vi "HW1 Calculator.vi"() -> ()   [LabVIEW 2023]
uses:
  <vilib>/gmath/NI_Gmath.lvlib
panel:
  in  "1/x":bool
  out "Save 2":ext
  out "Save1":ext
  in  "Save 2":bool
  in  "Save 1":bool
  out "Answer":ext
  out "運行時間":string
  in  "stop":bool
  out "Display":string
  in  ")":bool
  in  "(":bool
  in  "=":bool
  in  "+":bool
  in  ".":bool
  in  "+/-":bool
  in  "0":bool
  in  "Backspace":bool
  in  "CE":bool
  in  "C":bool
  in  "SQRT":bool
  in  "-":bool
  in  "*":bool
  in  "/":bool
  in  "9":bool
  in  "8":bool
  in  "7":bool
  in  "6":bool
  in  "5":bool
  in  "4":bool
  in  "3":bool
  in  "2":bool
  in  "1":bool
  out "current time":timestamp format="%<%I:%M:%S %p\n%x>T"
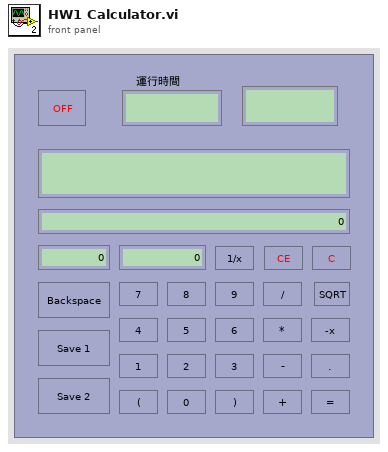
[diagram p1: front panel]
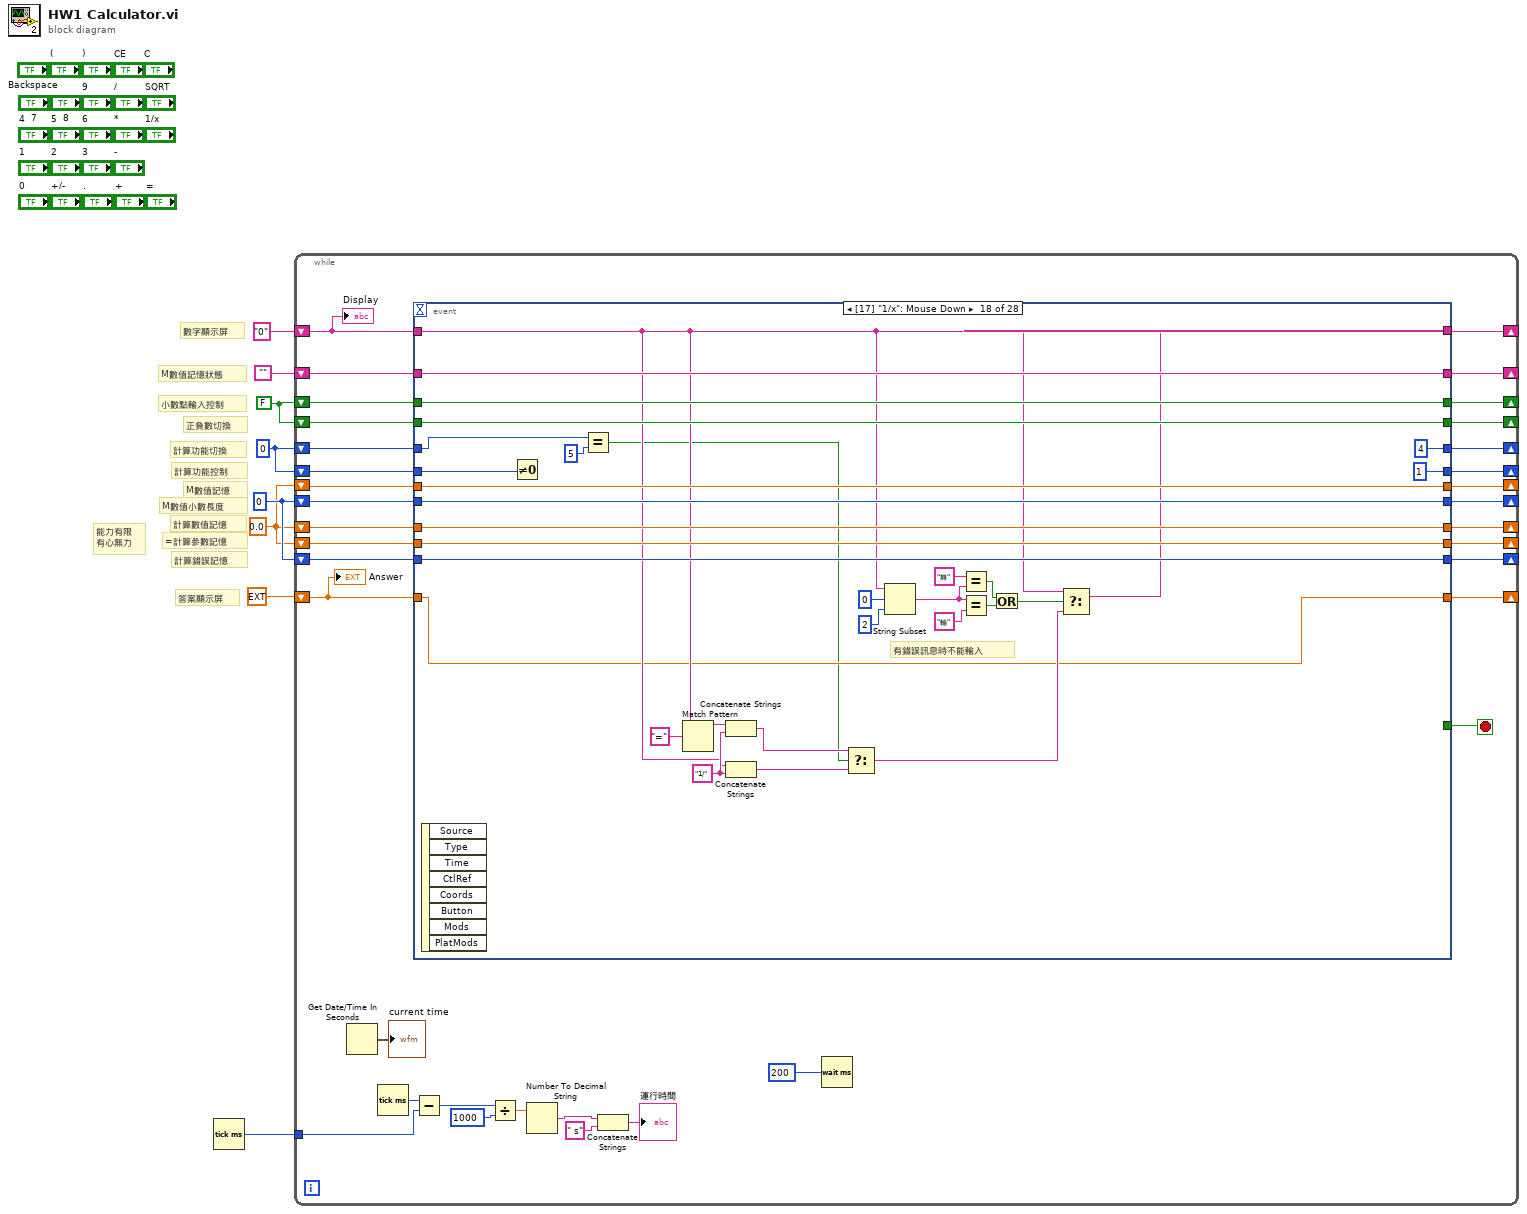
[diagram p0: block diagram]
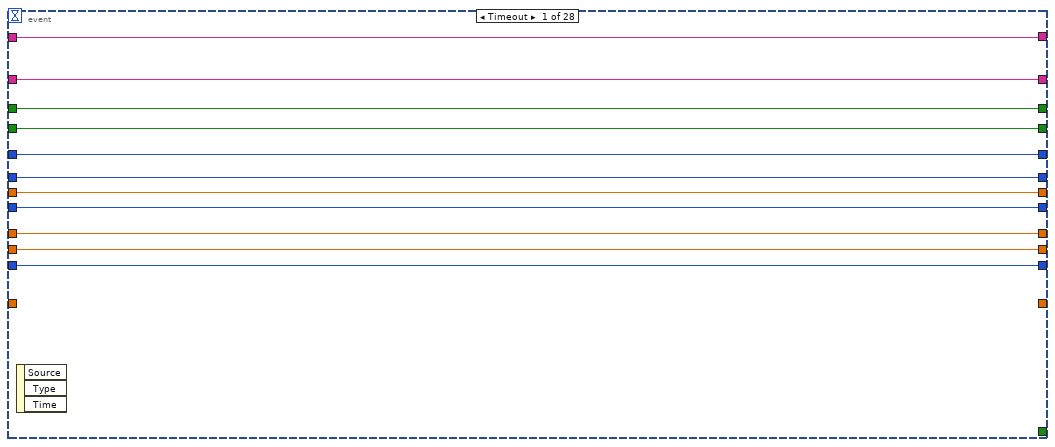
[diagram p2: hidden frame]
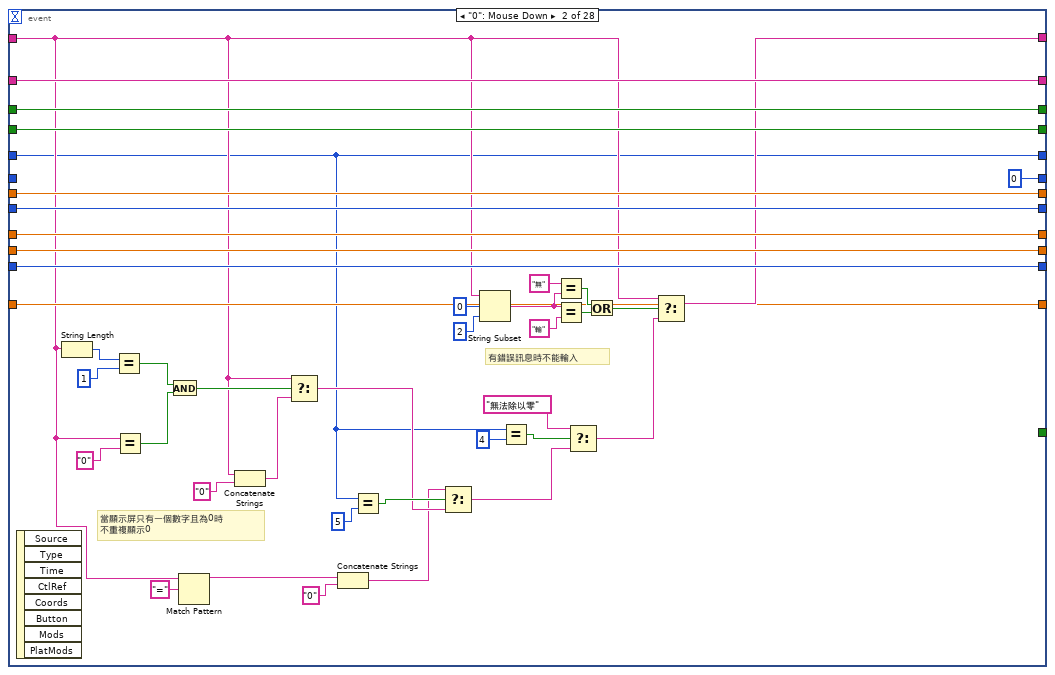
[diagram p3: hidden frame]
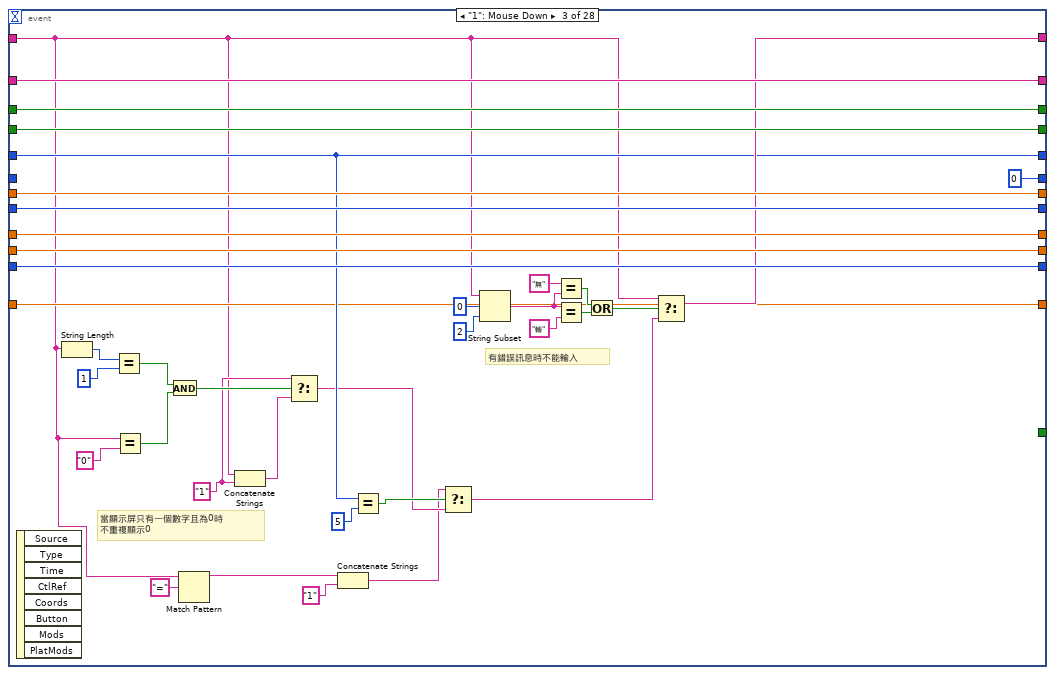
[diagram p4: hidden frame]
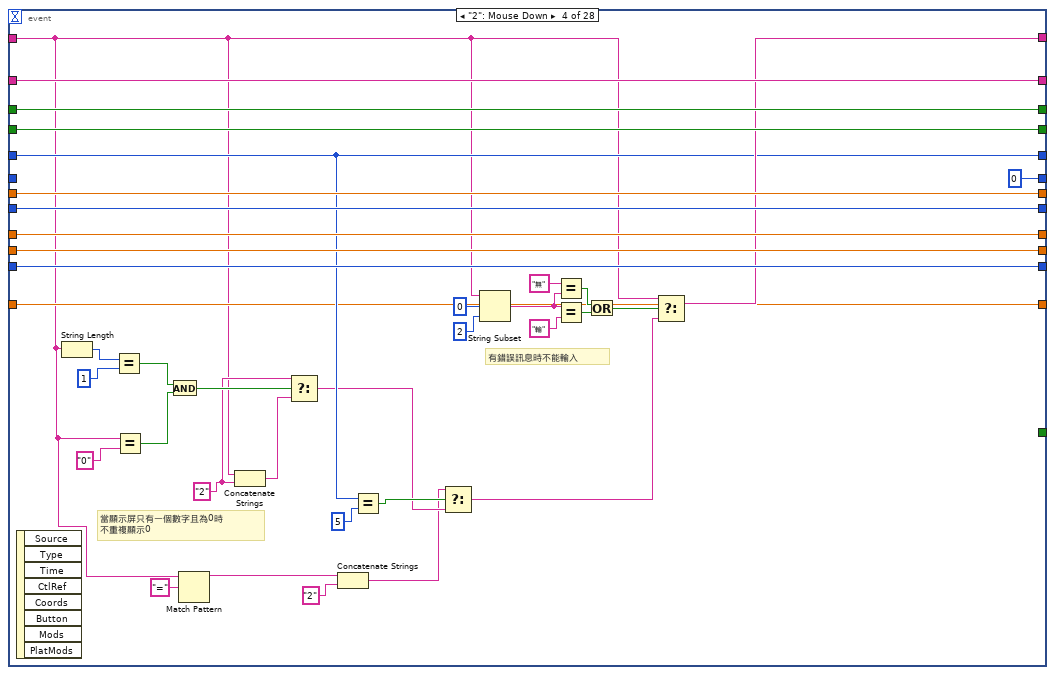
[diagram p5: hidden frame]
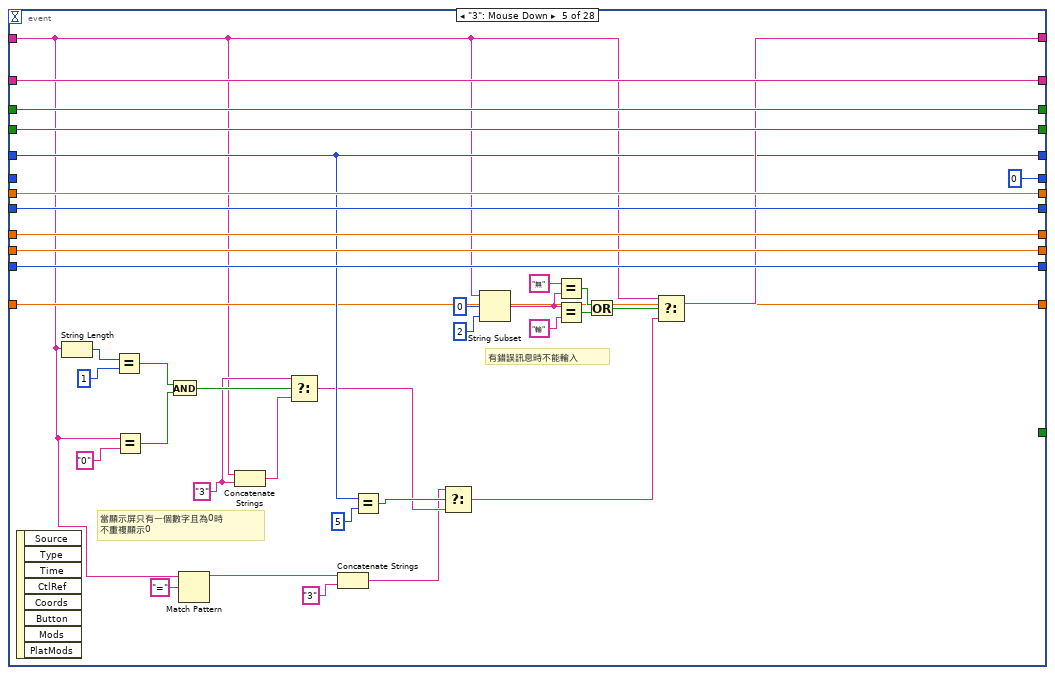
[diagram p6: hidden frame]
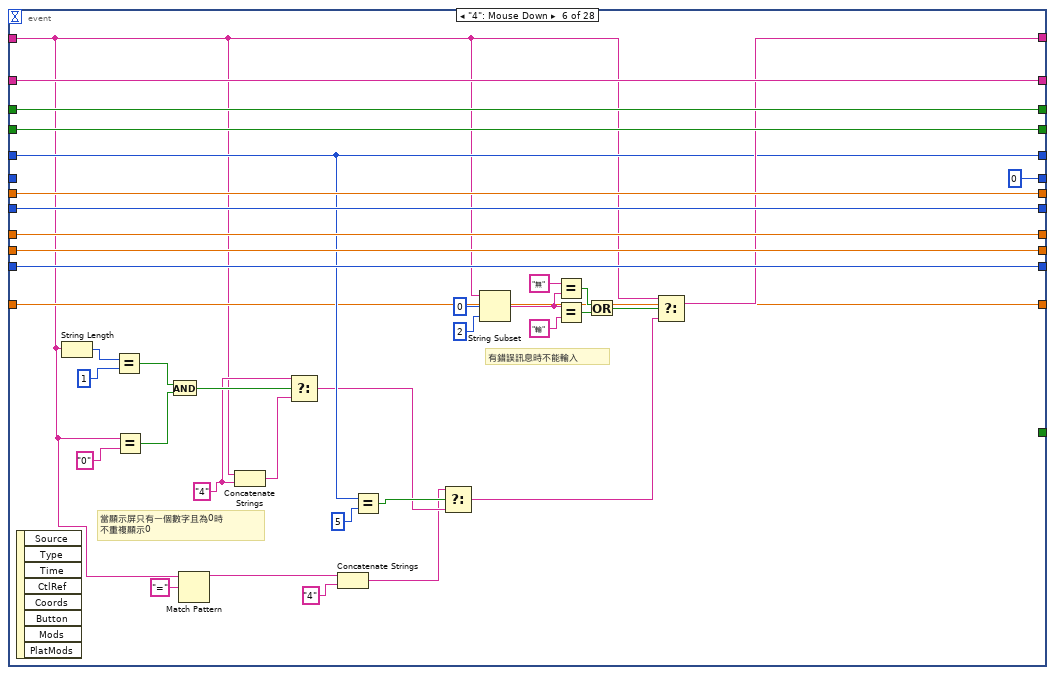
[diagram p7: hidden frame]
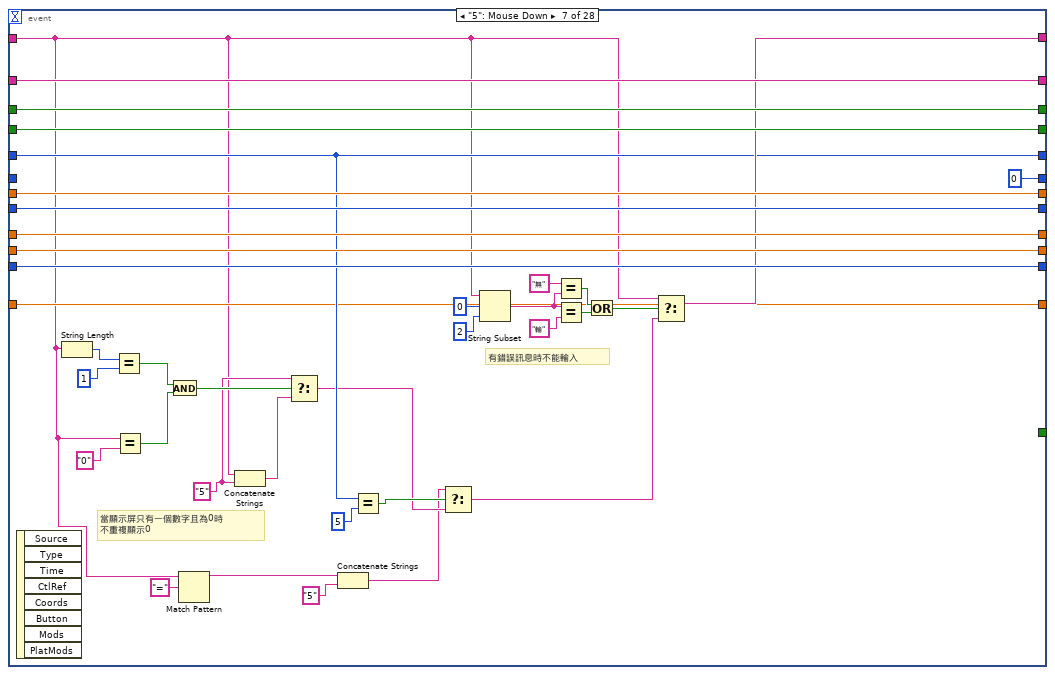
[diagram p8: hidden frame]
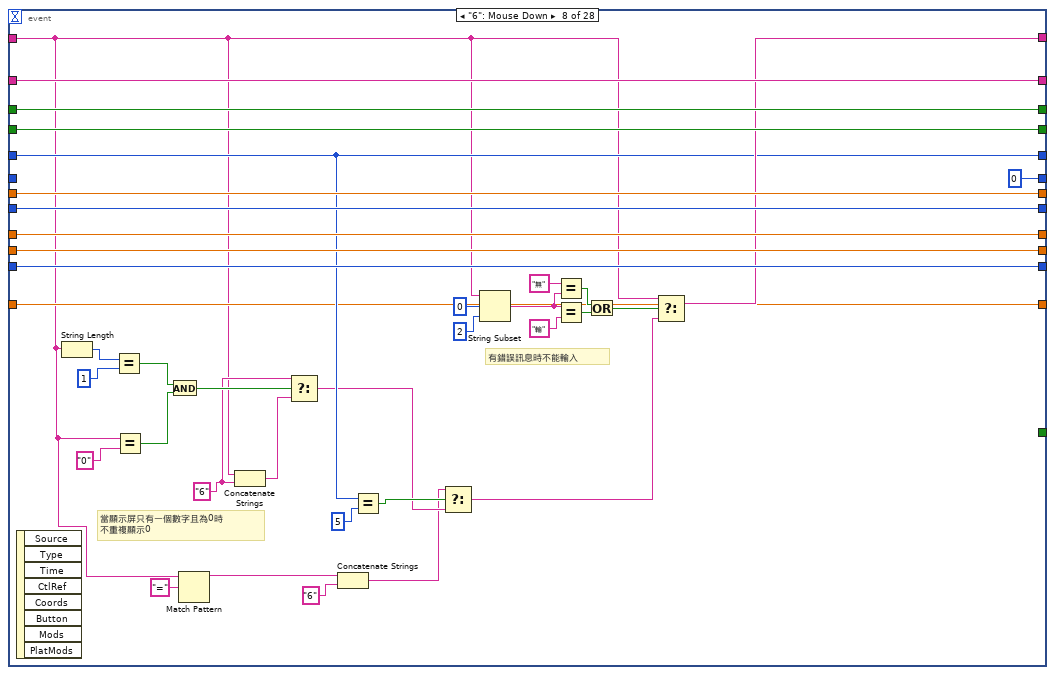
[diagram p9: hidden frame]
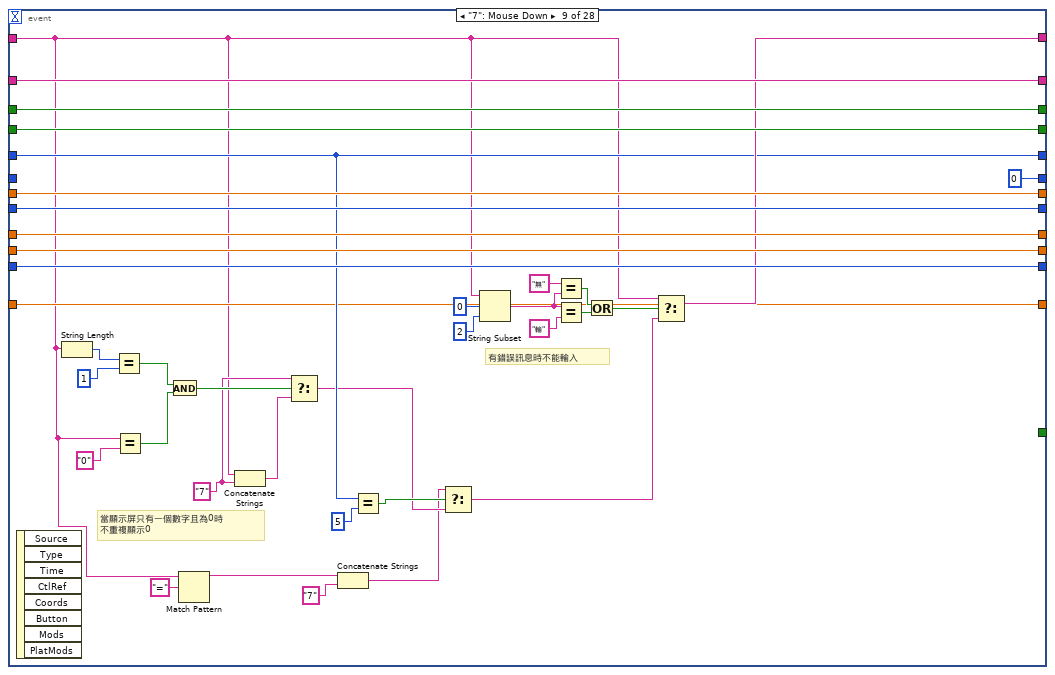
[diagram p10: hidden frame]
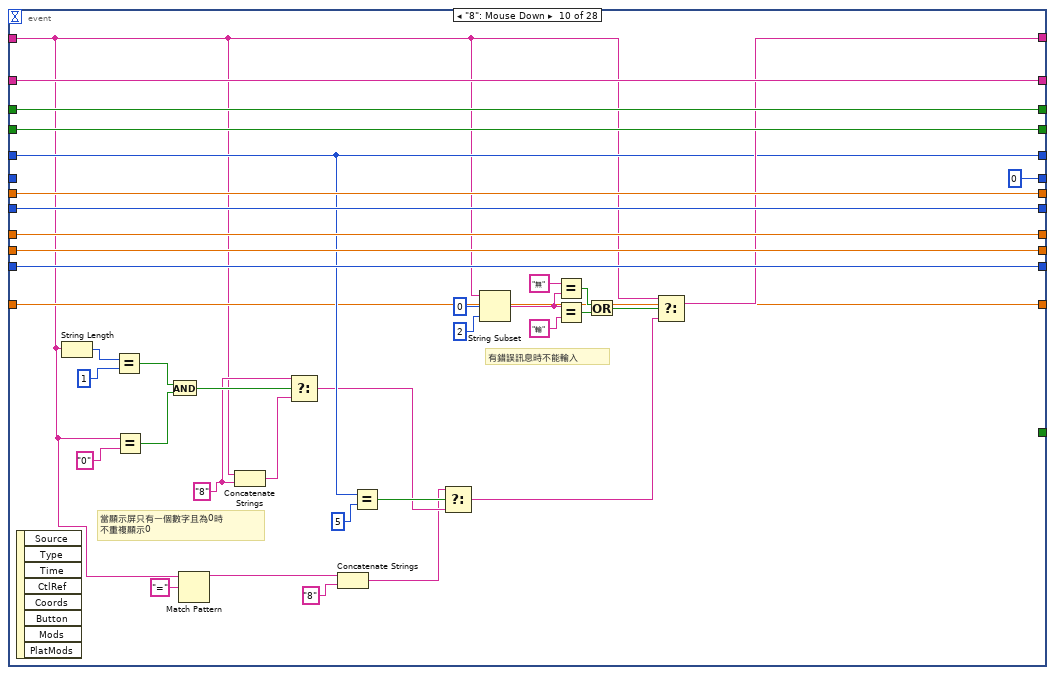
[diagram p11: hidden frame]
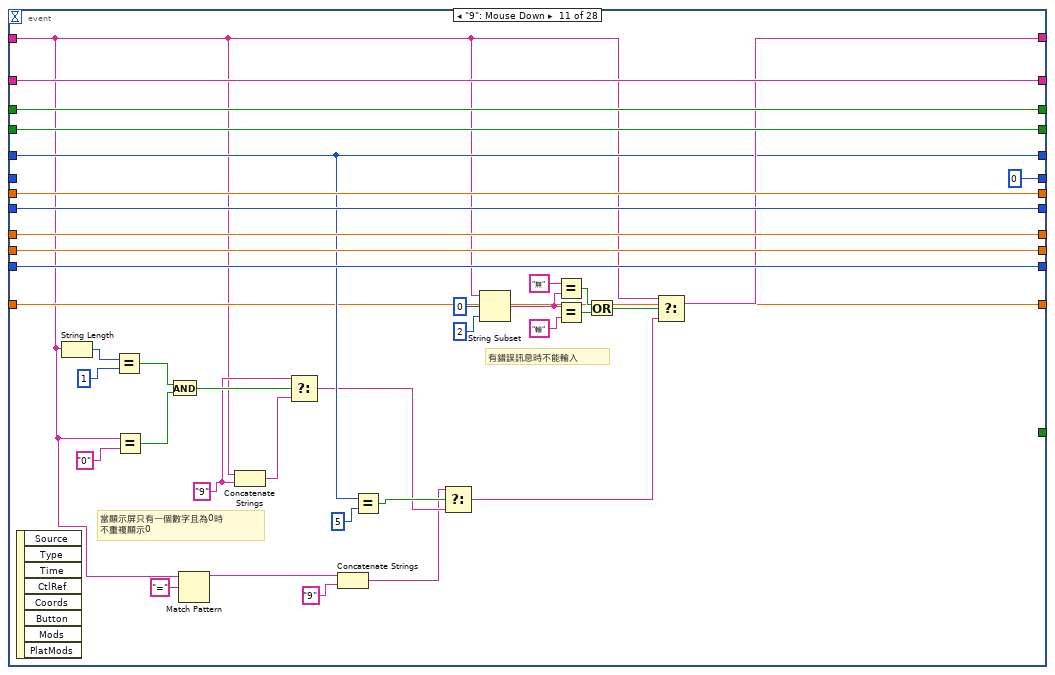
[diagram p12: hidden frame]
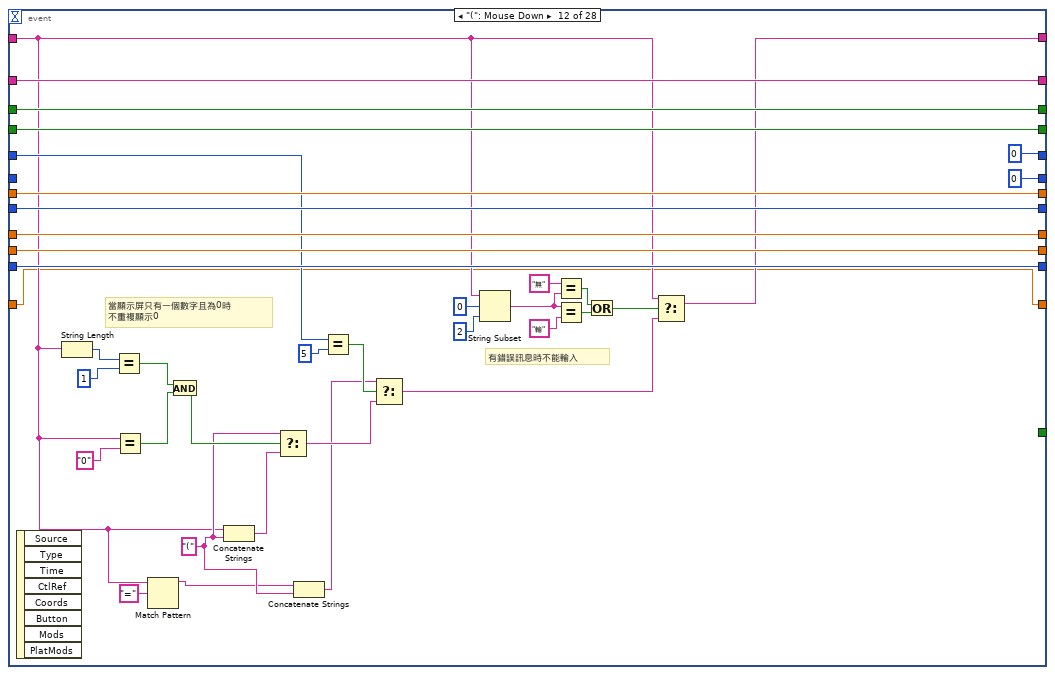
[diagram p13: hidden frame]
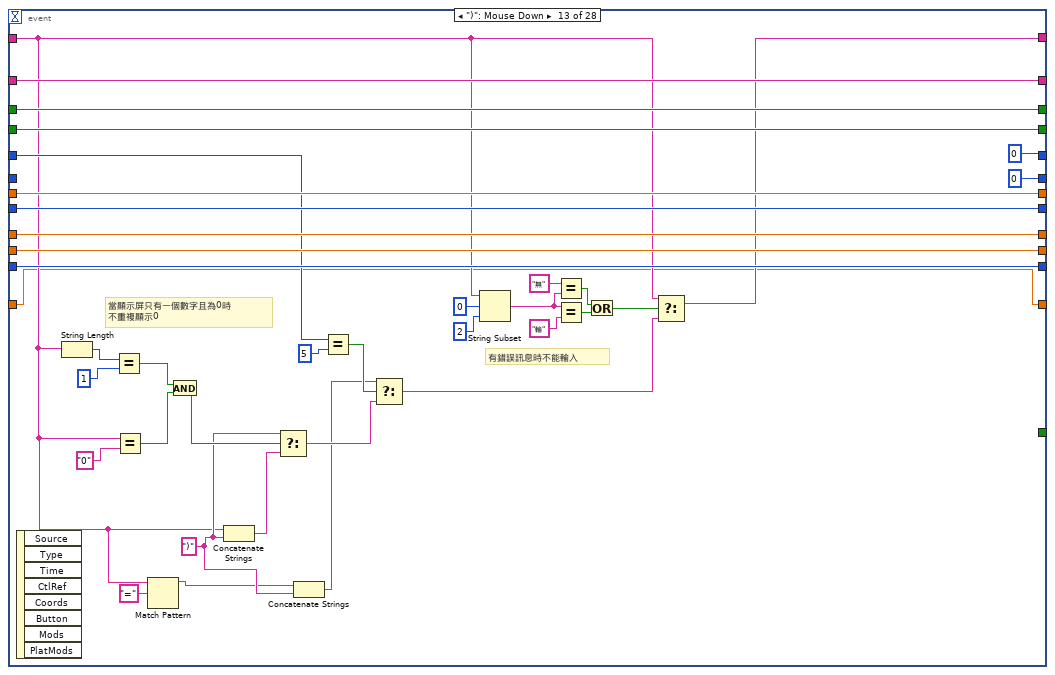
[diagram p14: hidden frame]
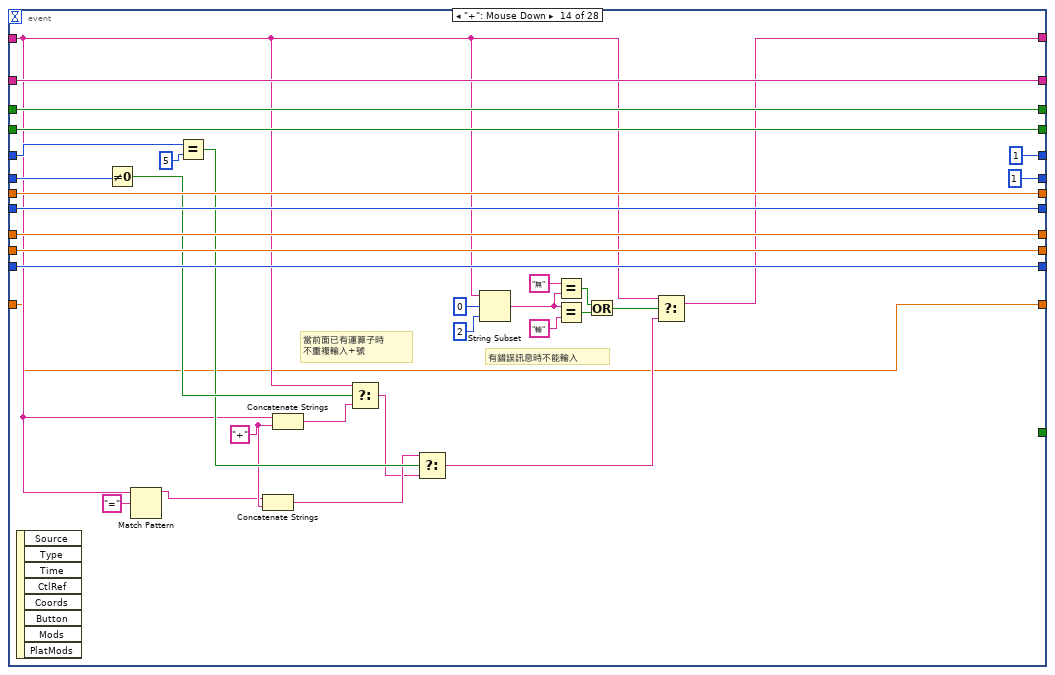
[diagram p15: hidden frame]
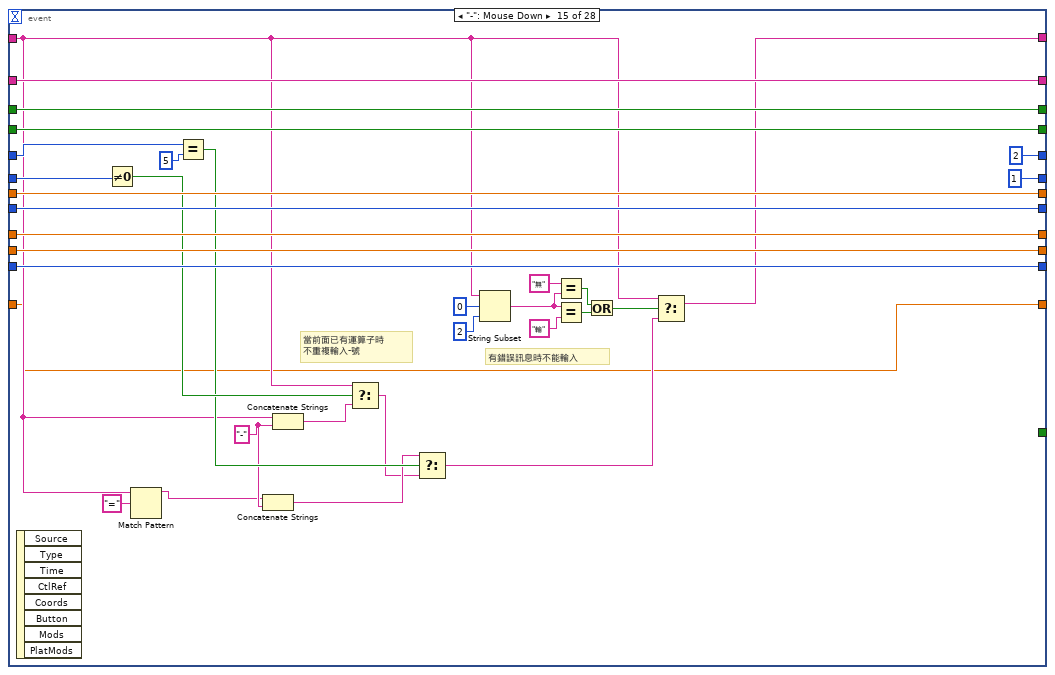
[diagram p16: hidden frame]
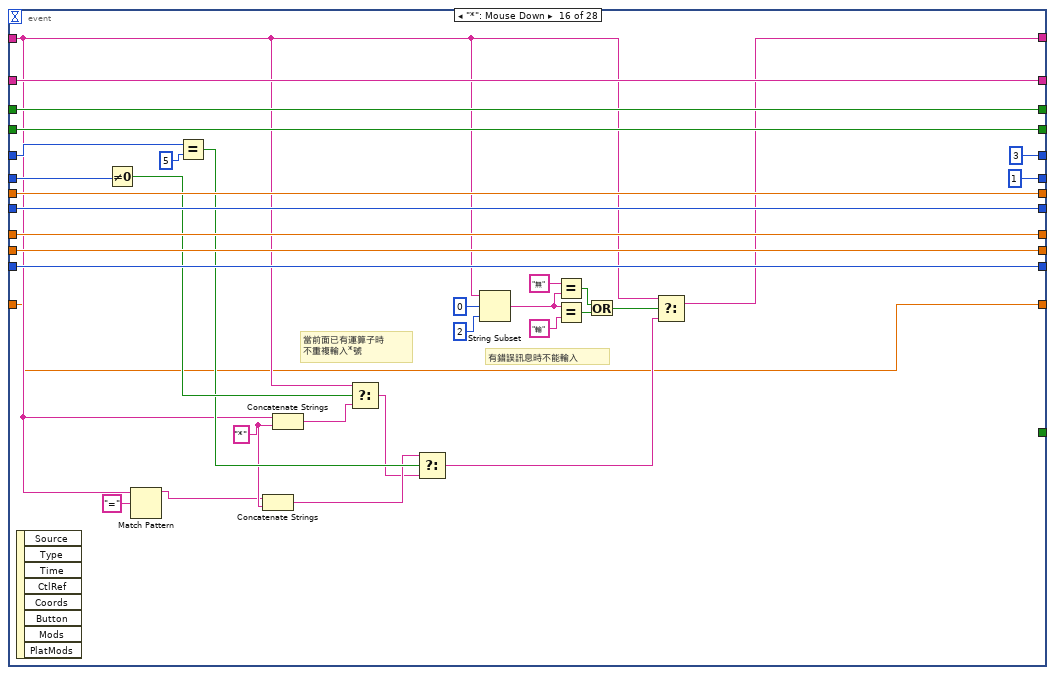
[diagram p17: hidden frame]
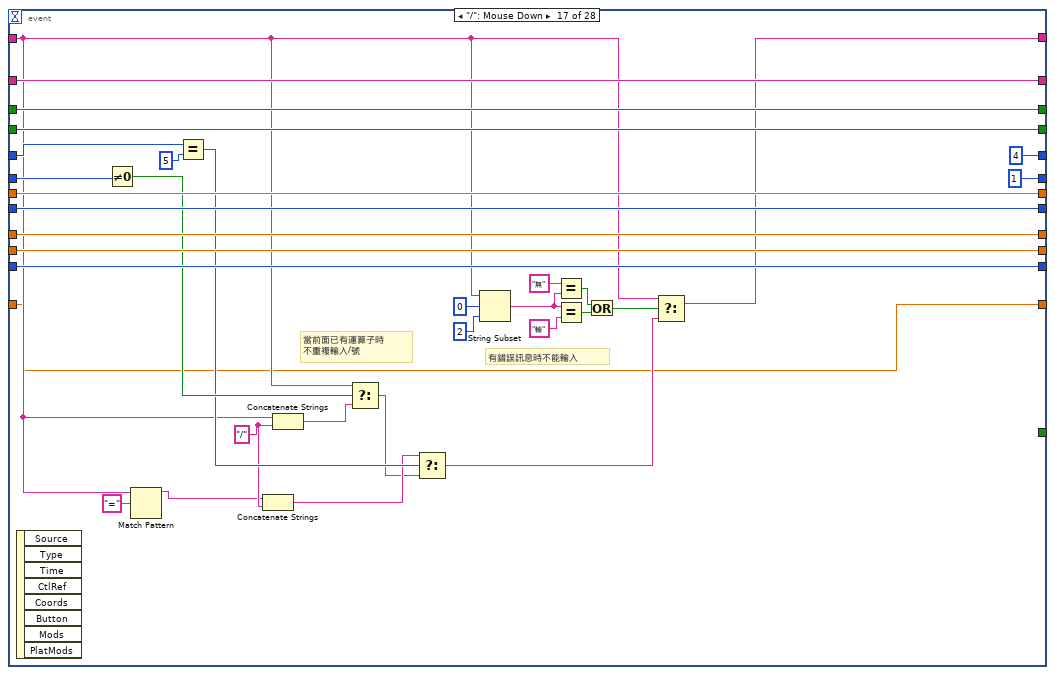
[diagram p18: hidden frame]
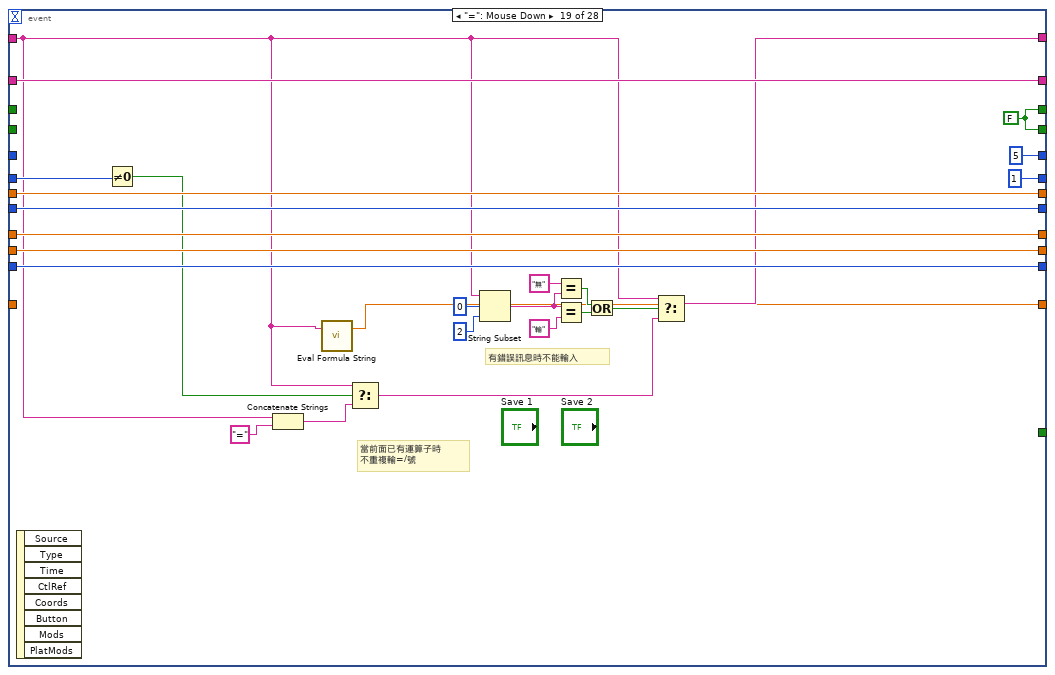
[diagram p19: hidden frame]
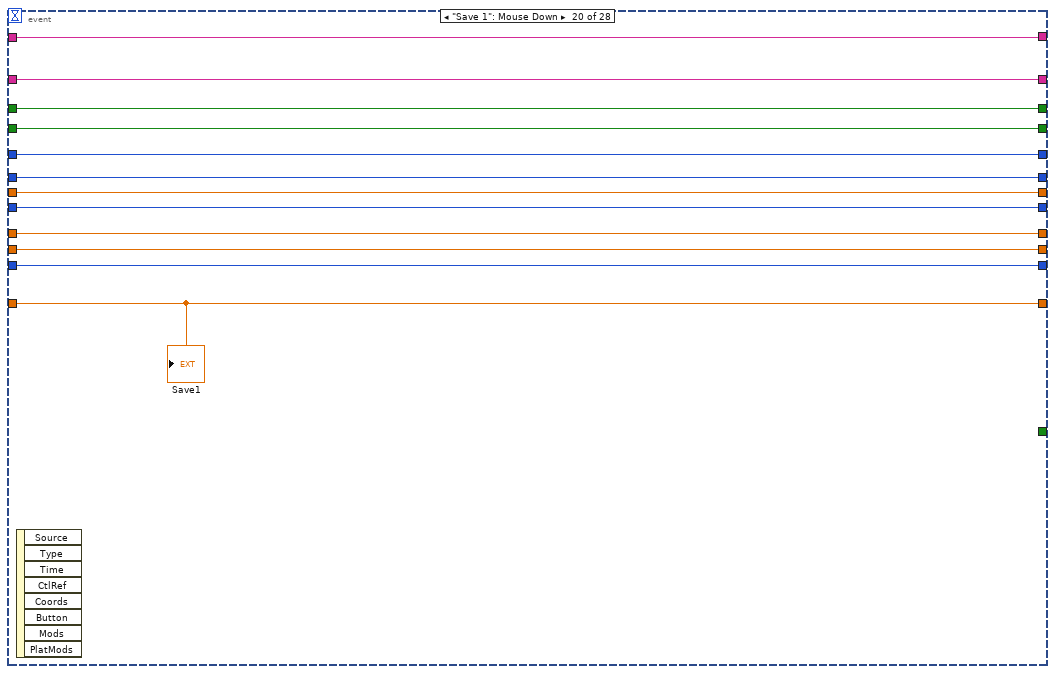
[diagram p20: hidden frame]
diagram:
  w3 = 0.0
  w4 = 0
  w5 = 0
  w6 = FALSE
  # "能力有限\n有心無力"
  # "答案顯示屏"
  # "M數值小數長度"
  # "計算錯誤記憶"
  # "=計算參數記憶"
  # "計算數值記憶"
  # "M數值記憶"
  # "計算功能控制"
  # "計算功能切換"
  # "正負數切換"
  # "小數點輸入控制"
  # "M數值記憶狀態"
  # "數字顯示屏"
  n1 = Tick Count (ms)() -> (millisecond timer value=w2:u32)
  n2 = while {
    shift-right: [w43] -> _
    shift-left: "0" -> [w24]
    shift-right: [w42] -> _
    shift-left: "" -> [w23]
    shift-right: [w40] -> _
    shift-left: w6 -> [w41]
    shift-right: [w38] -> _
    shift-left: w6 -> [w39]
    shift-right: [w37] -> _
    shift-left: w5 -> [w22]
    shift-right: [w35] -> _
    shift-left: w5 -> [w36]
    shift-right: [w27] -> _
    shift-left: w3 -> [w28]
    shift-right: [w33] -> _
    shift-left: w4 -> [w34]
    shift-right: [w29] -> _
    shift-left: w3 -> [w30]
    shift-right: [w25] -> _
    shift-left: w3 -> [w26]
    shift-right: [w31] -> _
    shift-left: w4 -> [w32]
    tunnel: w2 -> [w20]
    shift-right: [w12] -> _
    shift-left: ext 0.0 -> [w11]
    stop <- w21 stop-if-true
    n3 = Get Date/Time In Seconds() -> (seconds since 1Jan1904=→"current time":timestamp)
    n4 = Tick Count (ms)() -> (millisecond timer value=w19:u32)
    n5 = event shown="[17] \"1/x\": Mouse Down" {
      selector: _ -> [_ _ _ _ _ _ _ _ _ _ _ _ _ _ _ _ _ _ _ _ _ _ _ _ _ _ _ _]
      dyn-events: _ -> [_ _ _ _ _ _ _ _ _ _ _ _ _ _ _ _ _ _ _ _ _ _ _ _ _ _ _ _]
      timeout: _ -> [_ _ _ _ _ _ _ _ _ _ _ _ _ _ _ _ _ _ _ _ _ _ _ _ _ _ _ _]
      tunnel: w24 -> [w54 w64 w98 w135 w172 w209 w246 w283 w320 w357 w394 w432 w469 w506 w539 w572 w605 w640 w669 w702 w714 w724 w765 w802 _ w869 w881 _]
      tunnel: [w54 w70 w108 w145 w182 w219 w256 w293 w330 w367 w404 w441 w478 w518 w551 w584 w617 w648 w675 w702 w714 w740 w785 w824 "0" w868 w893 _] -> w43
      tunnel: w23 -> [w53 w95 w132 w169 w206 w243 w280 w317 w354 w391 w428 w465 w502 w535 w568 w601 w634 w665 w690 w701 w713 w760 w800 w839 w847 w874 w894 _]
      tunnel: [w53 w95 w132 w169 w206 w243 w280 w317 w354 w391 w428 w465 w502 w535 w568 w601 w634 w665 w690 w701 w713 w760 w800 w839 w847 w874 w894 _] -> w42
      tunnel: w41 -> [w52 w94 w131 w168 w205 w242 w279 w316 w353 w390 w427 w464 w501 w534 w567 w600 w633 w664 _ w700 w712 w759 w770 w810 _ w867 w896 _]
      tunnel: [w52 w94 w131 w168 w205 w242 w279 w316 w353 w390 w427 w464 w501 w534 w567 w600 w633 w664 w666 w700 w712 w759 w769 w820 w848 w866 w896 _] -> w40
      tunnel: w39 -> [w51 w93 w130 w167 w204 w241 w278 w315 w352 w389 w426 w463 w500 w533 w566 w599 w632 w663 _ w699 w711 w736 w774 w838 _ w864 w895 _]
      tunnel: [w51 w93 w130 w167 w204 w241 w278 w315 w352 w389 w426 w463 w500 w533 w566 w599 w632 w663 w666 w699 w711 w729 w768 w838 w848 w863 w895 _] -> w38
      tunnel: w22 -> [w50 w59 w106 w143 w180 w217 w254 w291 w328 w365 w402 w440 w477 w512 w545 w578 w611 w644 _ w698 w710 w721 _ w815 _ w861 w883 _]
      tunnel: [w50 w59 w106 w143 w180 w217 w254 w291 w328 w365 w402 0 0 1 2 3 4 4 5 w698 w710 0 0 0 w840 w859 w885 _] -> w37
      tunnel: w36 -> [w49 _ _ _ _ _ _ _ _ _ _ _ _ w517 w550 w583 w616 w647 w673 w697 w709 w734 w779 w819 _ w860 _ _]
      tunnel: [w49 0 0 0 0 0 0 0 0 0 0 0 0 1 1 1 1 1 1 w697 w709 0 w779 0 w840 w858 w885 _] -> w35
      tunnel: w34 -> [w48 w91 w128 w165 w202 w239 w276 w313 w350 w387 w424 w461 w498 w531 w564 w597 w630 w661 w688 w695 w707 w757 w798 w836 w845 w872 w911 _]
      tunnel: [w48 w91 w128 w165 w202 w239 w276 w313 w350 w387 w424 w461 w498 w531 w564 w597 w630 w661 w688 w695 w707 w757 w798 w836 w845 w872 w911 _] -> w33
      tunnel: w32 -> [w47 w88 w125 w162 w199 w236 w273 w310 w347 w384 w421 w458 w495 w528 w561 w594 w627 w658 w685 w692 w704 w754 w795 w833 w842 w853 w908 _]
      tunnel: [w47 w88 w125 w162 w199 w236 w273 w310 w347 w384 w421 w458 w495 w528 w561 w594 w627 w658 w685 w692 w704 w754 w795 w833 w842 w852 w908 _] -> w31
      tunnel: w30 -> [w46 w90 w127 w164 w201 w238 w275 w312 w349 w386 w423 w460 w497 w530 w563 w596 w629 w660 w687 w694 w706 w756 w797 w835 w844 w856 w910 _]
      tunnel: [w46 w90 w127 w164 w201 w238 w275 w312 w349 w386 w423 w460 w497 w530 w563 w596 w629 w660 w687 w694 w706 w756 w797 w835 w844 w854 w910 _] -> w29
      tunnel: w28 -> [w45 w92 w129 w166 w203 w240 w277 w314 w351 w388 w425 w462 w499 w532 w565 w598 w631 w662 w689 w696 w708 w758 w799 w837 w846 w873 w912 _]
      tunnel: [w45 w92 w129 w166 w203 w240 w277 w314 w351 w388 w425 w462 w499 w532 w565 w598 w631 w662 w689 w696 w708 w758 w799 w837 w846 w873 w912 _] -> w27
      tunnel: w26 -> [w44 w89 w126 w163 w200 w237 w274 w311 w348 w385 w422 w459 w496 w529 w562 w595 w628 w659 w686 w693 w705 w755 w796 w834 w843 w855 w909 _]
      tunnel: [w44 w89 w126 w163 w200 w237 w274 w311 w348 w385 w422 w459 w496 w529 w562 w595 w628 w659 w686 w693 w705 w755 w796 w834 w843 w850 w909 _] -> w25
      tunnel: [_ _ _ _ _ _ _ _ _ _ _ _ _ _ _ _ _ _ _ _ _ _ _ _ _ _ _ w913] -> w21
      tunnel: [_ w65 w100 w137 w174 w211 w248 w285 w322 w359 w396 w429 w466 w503 w536 w569 w602 w637 w667 w691 w703 _ w761 _ w841 w850 w876 _] -> w12
      tunnel: w11 -> [_ w65 w100 w137 w174 w211 w248 w285 w322 w359 w396 w429 w466 w503 w536 w569 w602 w637 _ w691 w703 w719 w761 _ w841 _ w876 _]
      event Timeout {
        n6 = event-data() -> ()  [unwired: 1 in, 3 out]
      }
      event "0": Mouse Down {
        # "有錯誤訊息時不能輸入"
        # "當顯示屏只有一個數字且為0時\n不重複顯示0"
        n7 = event-data() -> ()  [unwired: 1 in, 8 out]
        n8 = String Length(string=w64) -> (length=w85:i32)
        n9 = Equal?(x=w85, y=1) -> (x = y?=w83:bool)
        n10 = Equal?(x=w64, y="0") -> (x = y?=w82:bool)
        n11 = And(x=w83, y=w82) -> (x .and. y?=w80:bool)
        n12 = Match Pattern(string=w64, regular expression="=") -> (before substring=w62:string)  [unwired: 1 in, 3 out]
        n13 = Concatenate Strings(w64, "0") -> (w79:string)
        n14 = Select(t=w64, s=w80, f=w79) -> (s? t:f=w67:string)
        n15 = Concatenate Strings(w62, "0") -> (w61:string)
        n16 = Equal?(x=w59, y=5) -> (x = y?=w68:bool)
        n17 = Select(t=w61, s=w68, f=w67) -> (s? t:f=w58:string)
        n18 = String Subset(string=w64, offset (0)=0, length (rest)=2) -> (substring=w74:string)
        n19 = Equal?(x=w59, y=4) -> (x = y?=w57:bool)
        n20 = Equal?(x="無", y=w74) -> (x = y?=w73:bool)
        n21 = Equal?(x=w74, y="輸") -> (x = y?=w72:bool)
        n22 = Select(t="無法除以零", s=w57, f=w58) -> (s? t:f=w55:string)
        n23 = Or(x=w73, y=w72) -> (x .or. y?=w71:bool)
        n24 = Select(t=w64, s=w71, f=w55) -> (s? t:f=w70:string)
      }
      event "1": Mouse Down {
        w99 = "1"
        # "有錯誤訊息時不能輸入"
        # "當顯示屏只有一個數字且為0時\n不重複顯示0"
        n25 = event-data() -> ()  [unwired: 1 in, 8 out]
        n26 = String Length(string=w98) -> (length=w122:i32)
        n27 = Equal?(x=w122, y=1) -> (x = y?=w120:bool)
        n28 = Equal?(x=w98, y="0") -> (x = y?=w119:bool)
        n29 = And(x=w120, y=w119) -> (x .and. y?=w118:bool)
        n30 = Match Pattern(string=w98, regular expression="=") -> (before substring=w96:string)  [unwired: 1 in, 3 out]
        n31 = Concatenate Strings(w98, w99) -> (w117:string)
        n32 = Select(t=w99, s=w118, f=w117) -> (s? t:f=w104:string)
        n33 = Concatenate Strings(w96, "1") -> (w102:string)
        n34 = Equal?(x=w106, y=5) -> (x = y?=w105:bool)
        n35 = Select(t=w102, s=w105, f=w104) -> (s? t:f=w101:string)
        n36 = String Subset(string=w98, offset (0)=0, length (rest)=2) -> (substring=w112:string)
        n37 = Equal?(x="無", y=w112) -> (x = y?=w111:bool)
        n38 = Equal?(x=w112, y="輸") -> (x = y?=w110:bool)
        n39 = Or(x=w111, y=w110) -> (x .or. y?=w109:bool)
        n40 = Select(t=w98, s=w109, f=w101) -> (s? t:f=w108:string)
      }
      event "2": Mouse Down {
        w136 = "2"
        # "有錯誤訊息時不能輸入"
        # "當顯示屏只有一個數字且為0時\n不重複顯示0"
        n41 = event-data() -> ()  [unwired: 1 in, 8 out]
        n42 = String Length(string=w135) -> (length=w159:i32)
        n43 = Equal?(x=w159, y=1) -> (x = y?=w157:bool)
        n44 = Equal?(x=w135, y="0") -> (x = y?=w156:bool)
        n45 = And(x=w157, y=w156) -> (x .and. y?=w155:bool)
        n46 = Match Pattern(string=w135, regular expression="=") -> (before substring=w133:string)  [unwired: 1 in, 3 out]
        n47 = Concatenate Strings(w135, w136) -> (w154:string)
        n48 = Select(t=w136, s=w155, f=w154) -> (s? t:f=w141:string)
        n49 = Concatenate Strings(w133, "2") -> (w139:string)
        n50 = Equal?(x=w143, y=5) -> (x = y?=w142:bool)
        n51 = Select(t=w139, s=w142, f=w141) -> (s? t:f=w138:string)
        n52 = String Subset(string=w135, offset (0)=0, length (rest)=2) -> (substring=w149:string)
        n53 = Equal?(x="無", y=w149) -> (x = y?=w148:bool)
        n54 = Equal?(x=w149, y="輸") -> (x = y?=w147:bool)
        n55 = Or(x=w148, y=w147) -> (x .or. y?=w146:bool)
        n56 = Select(t=w135, s=w146, f=w138) -> (s? t:f=w145:string)
      }
      event "3": Mouse Down {
        w173 = "3"
        # "有錯誤訊息時不能輸入"
        # "當顯示屏只有一個數字且為0時\n不重複顯示0"
        n57 = event-data() -> ()  [unwired: 1 in, 8 out]
        n58 = String Length(string=w172) -> (length=w196:i32)
        n59 = Equal?(x=w196, y=1) -> (x = y?=w194:bool)
        n60 = Equal?(x=w172, y="0") -> (x = y?=w193:bool)
        n61 = And(x=w194, y=w193) -> (x .and. y?=w192:bool)
        n62 = Match Pattern(string=w172, regular expression="=") -> (before substring=w170:string)  [unwired: 1 in, 3 out]
        n63 = Concatenate Strings(w172, w173) -> (w191:string)
        n64 = Select(t=w173, s=w192, f=w191) -> (s? t:f=w178:string)
        n65 = Concatenate Strings(w170, "3") -> (w176:string)
        n66 = Equal?(x=w180, y=5) -> (x = y?=w179:bool)
        n67 = Select(t=w176, s=w179, f=w178) -> (s? t:f=w175:string)
        n68 = String Subset(string=w172, offset (0)=0, length (rest)=2) -> (substring=w186:string)
        n69 = Equal?(x="無", y=w186) -> (x = y?=w185:bool)
        n70 = Equal?(x=w186, y="輸") -> (x = y?=w184:bool)
        n71 = Or(x=w185, y=w184) -> (x .or. y?=w183:bool)
        n72 = Select(t=w172, s=w183, f=w175) -> (s? t:f=w182:string)
      }
      event "4": Mouse Down {
        w210 = "4"
        # "有錯誤訊息時不能輸入"
        # "當顯示屏只有一個數字且為0時\n不重複顯示0"
        n73 = event-data() -> ()  [unwired: 1 in, 8 out]
        n74 = String Length(string=w209) -> (length=w233:i32)
        n75 = Equal?(x=w233, y=1) -> (x = y?=w231:bool)
        n76 = Equal?(x=w209, y="0") -> (x = y?=w230:bool)
        n77 = And(x=w231, y=w230) -> (x .and. y?=w229:bool)
        n78 = Match Pattern(string=w209, regular expression="=") -> (before substring=w207:string)  [unwired: 1 in, 3 out]
        n79 = Concatenate Strings(w209, w210) -> (w228:string)
        n80 = Select(t=w210, s=w229, f=w228) -> (s? t:f=w215:string)
        n81 = Concatenate Strings(w207, "4") -> (w213:string)
        n82 = Equal?(x=w217, y=5) -> (x = y?=w216:bool)
        n83 = Select(t=w213, s=w216, f=w215) -> (s? t:f=w212:string)
        n84 = String Subset(string=w209, offset (0)=0, length (rest)=2) -> (substring=w223:string)
        n85 = Equal?(x="無", y=w223) -> (x = y?=w222:bool)
        n86 = Equal?(x=w223, y="輸") -> (x = y?=w221:bool)
        n87 = Or(x=w222, y=w221) -> (x .or. y?=w220:bool)
        n88 = Select(t=w209, s=w220, f=w212) -> (s? t:f=w219:string)
      }
      event "5": Mouse Down {
        w247 = "5"
        # "有錯誤訊息時不能輸入"
        # "當顯示屏只有一個數字且為0時\n不重複顯示0"
        n89 = event-data() -> ()  [unwired: 1 in, 8 out]
        n90 = String Length(string=w246) -> (length=w270:i32)
        n91 = Equal?(x=w270, y=1) -> (x = y?=w268:bool)
        n92 = Equal?(x=w246, y="0") -> (x = y?=w267:bool)
        n93 = And(x=w268, y=w267) -> (x .and. y?=w266:bool)
        n94 = Match Pattern(string=w246, regular expression="=") -> (before substring=w244:string)  [unwired: 1 in, 3 out]
        n95 = Concatenate Strings(w246, w247) -> (w265:string)
        n96 = Select(t=w247, s=w266, f=w265) -> (s? t:f=w252:string)
        n97 = Concatenate Strings(w244, "5") -> (w250:string)
        n98 = Equal?(x=w254, y=5) -> (x = y?=w253:bool)
        n99 = Select(t=w250, s=w253, f=w252) -> (s? t:f=w249:string)
        n100 = String Subset(string=w246, offset (0)=0, length (rest)=2) -> (substring=w260:string)
        n101 = Equal?(x="無", y=w260) -> (x = y?=w259:bool)
        n102 = Equal?(x=w260, y="輸") -> (x = y?=w258:bool)
        n103 = Or(x=w259, y=w258) -> (x .or. y?=w257:bool)
        n104 = Select(t=w246, s=w257, f=w249) -> (s? t:f=w256:string)
      }
      event "6": Mouse Down {
        w284 = "6"
        # "有錯誤訊息時不能輸入"
        # "當顯示屏只有一個數字且為0時\n不重複顯示0"
        n105 = event-data() -> ()  [unwired: 1 in, 8 out]
        n106 = String Length(string=w283) -> (length=w307:i32)
        n107 = Equal?(x=w307, y=1) -> (x = y?=w305:bool)
        n108 = Equal?(x=w283, y="0") -> (x = y?=w304:bool)
        n109 = And(x=w305, y=w304) -> (x .and. y?=w303:bool)
        n110 = Match Pattern(string=w283, regular expression="=") -> (before substring=w281:string)  [unwired: 1 in, 3 out]
        n111 = Concatenate Strings(w283, w284) -> (w302:string)
        n112 = Select(t=w284, s=w303, f=w302) -> (s? t:f=w289:string)
        n113 = Concatenate Strings(w281, "6") -> (w287:string)
        n114 = Equal?(x=w291, y=5) -> (x = y?=w290:bool)
        n115 = Select(t=w287, s=w290, f=w289) -> (s? t:f=w286:string)
        n116 = String Subset(string=w283, offset (0)=0, length (rest)=2) -> (substring=w297:string)
        n117 = Equal?(x="無", y=w297) -> (x = y?=w296:bool)
        n118 = Equal?(x=w297, y="輸") -> (x = y?=w295:bool)
        n119 = Or(x=w296, y=w295) -> (x .or. y?=w294:bool)
        n120 = Select(t=w283, s=w294, f=w286) -> (s? t:f=w293:string)
      }
      event "7": Mouse Down {
        w321 = "7"
        # "有錯誤訊息時不能輸入"
        # "當顯示屏只有一個數字且為0時\n不重複顯示0"
        n121 = event-data() -> ()  [unwired: 1 in, 8 out]
        n122 = String Length(string=w320) -> (length=w344:i32)
        n123 = Equal?(x=w344, y=1) -> (x = y?=w342:bool)
        n124 = Equal?(x=w320, y="0") -> (x = y?=w341:bool)
        n125 = And(x=w342, y=w341) -> (x .and. y?=w340:bool)
        n126 = Match Pattern(string=w320, regular expression="=") -> (before substring=w318:string)  [unwired: 1 in, 3 out]
        n127 = Concatenate Strings(w320, w321) -> (w339:string)
        n128 = Select(t=w321, s=w340, f=w339) -> (s? t:f=w326:string)
        n129 = Concatenate Strings(w318, "7") -> (w324:string)
        n130 = Equal?(x=w328, y=5) -> (x = y?=w327:bool)
        n131 = Select(t=w324, s=w327, f=w326) -> (s? t:f=w323:string)
        n132 = String Subset(string=w320, offset (0)=0, length (rest)=2) -> (substring=w334:string)
        n133 = Equal?(x="無", y=w334) -> (x = y?=w333:bool)
        n134 = Equal?(x=w334, y="輸") -> (x = y?=w332:bool)
        n135 = Or(x=w333, y=w332) -> (x .or. y?=w331:bool)
        n136 = Select(t=w320, s=w331, f=w323) -> (s? t:f=w330:string)
      }
      event "8": Mouse Down {
        w358 = "8"
        # "有錯誤訊息時不能輸入"
        # "當顯示屏只有一個數字且為0時\n不重複顯示0"
        n137 = event-data() -> ()  [unwired: 1 in, 8 out]
        n138 = String Length(string=w357) -> (length=w381:i32)
        n139 = Equal?(x=w381, y=1) -> (x = y?=w379:bool)
        n140 = Equal?(x=w357, y="0") -> (x = y?=w378:bool)
        n141 = And(x=w379, y=w378) -> (x .and. y?=w377:bool)
        n142 = Match Pattern(string=w357, regular expression="=") -> (before substring=w355:string)  [unwired: 1 in, 3 out]
        n143 = Concatenate Strings(w357, w358) -> (w376:string)
        n144 = Select(t=w358, s=w377, f=w376) -> (s? t:f=w363:string)
        n145 = Concatenate Strings(w355, "8") -> (w361:string)
        n146 = Equal?(x=w365, y=5) -> (x = y?=w364:bool)
        n147 = Select(t=w361, s=w364, f=w363) -> (s? t:f=w360:string)
        n148 = String Subset(string=w357, offset (0)=0, length (rest)=2) -> (substring=w371:string)
        n149 = Equal?(x="無", y=w371) -> (x = y?=w370:bool)
        n150 = Equal?(x=w371, y="輸") -> (x = y?=w369:bool)
        n151 = Or(x=w370, y=w369) -> (x .or. y?=w368:bool)
        n152 = Select(t=w357, s=w368, f=w360) -> (s? t:f=w367:string)
      }
      event "9": Mouse Down {
        w395 = "9"
        # "有錯誤訊息時不能輸入"
        # "當顯示屏只有一個數字且為0時\n不重複顯示0"
        n153 = event-data() -> ()  [unwired: 1 in, 8 out]
        n154 = String Length(string=w394) -> (length=w418:i32)
        n155 = Equal?(x=w418, y=1) -> (x = y?=w416:bool)
        n156 = Equal?(x=w394, y="0") -> (x = y?=w415:bool)
        n157 = And(x=w416, y=w415) -> (x .and. y?=w414:bool)
        n158 = Match Pattern(string=w394, regular expression="=") -> (before substring=w392:string)  [unwired: 1 in, 3 out]
        n159 = Concatenate Strings(w394, w395) -> (w413:string)
        n160 = Select(t=w395, s=w414, f=w413) -> (s? t:f=w400:string)
        n161 = Concatenate Strings(w392, "9") -> (w398:string)
        n162 = Equal?(x=w402, y=5) -> (x = y?=w401:bool)
        n163 = Select(t=w398, s=w401, f=w400) -> (s? t:f=w397:string)
        n164 = String Subset(string=w394, offset (0)=0, length (rest)=2) -> (substring=w408:string)
        n165 = Equal?(x="無", y=w408) -> (x = y?=w407:bool)
        n166 = Equal?(x=w408, y="輸") -> (x = y?=w406:bool)
        n167 = Or(x=w407, y=w406) -> (x .or. y?=w405:bool)
        n168 = Select(t=w394, s=w405, f=w397) -> (s? t:f=w404:string)
      }
      event "(": Mouse Down {
        w436 = "("
        # "有錯誤訊息時不能輸入"
        # "當顯示屏只有一個數字且為0時\n不重複顯示0"
        n169 = event-data() -> ()  [unwired: 1 in, 8 out]
        n170 = String Length(string=w432) -> (length=w455:i32)
        n171 = Equal?(x=w455, y=1) -> (x = y?=w453:bool)
        n172 = Equal?(x=w432, y="0") -> (x = y?=w452:bool)
        n173 = Match Pattern(string=w432, regular expression="=") -> (before substring=w430:string)  [unwired: 1 in, 3 out]
        n174 = And(x=w453, y=w452) -> (x .and. y?=w451:bool)
        n175 = Concatenate Strings(w432, w436) -> (w450:string)
        n176 = Select(t=w436, s=w451, f=w450) -> (s? t:f=w437:string)
        n177 = Concatenate Strings(w430, w436) -> (w435:string)
        n178 = Equal?(x=w440, y=5) -> (x = y?=w438:bool)
        n179 = Select(t=w435, s=w438, f=w437) -> (s? t:f=w434:string)
        n180 = String Subset(string=w432, offset (0)=0, length (rest)=2) -> (substring=w445:string)
        n181 = Equal?(x="無", y=w445) -> (x = y?=w444:bool)
        n182 = Equal?(x=w445, y="輸") -> (x = y?=w443:bool)
        n183 = Or(x=w444, y=w443) -> (x .or. y?=w442:bool)
        n184 = Select(t=w432, s=w442, f=w434) -> (s? t:f=w441:string)
      }
      event ")": Mouse Down {
        w473 = ")"
        # "有錯誤訊息時不能輸入"
        # "當顯示屏只有一個數字且為0時\n不重複顯示0"
        n185 = event-data() -> ()  [unwired: 1 in, 8 out]
        n186 = String Length(string=w469) -> (length=w492:i32)
        n187 = Equal?(x=w492, y=1) -> (x = y?=w490:bool)
        n188 = Equal?(x=w469, y="0") -> (x = y?=w489:bool)
        n189 = Match Pattern(string=w469, regular expression="=") -> (before substring=w467:string)  [unwired: 1 in, 3 out]
        n190 = And(x=w490, y=w489) -> (x .and. y?=w488:bool)
        n191 = Concatenate Strings(w469, w473) -> (w487:string)
        n192 = Select(t=w473, s=w488, f=w487) -> (s? t:f=w474:string)
        n193 = Concatenate Strings(w467, w473) -> (w472:string)
        n194 = Equal?(x=w477, y=5) -> (x = y?=w475:bool)
        n195 = Select(t=w472, s=w475, f=w474) -> (s? t:f=w471:string)
        n196 = String Subset(string=w469, offset (0)=0, length (rest)=2) -> (substring=w482:string)
        n197 = Equal?(x="無", y=w482) -> (x = y?=w481:bool)
        n198 = Equal?(x=w482, y="輸") -> (x = y?=w480:bool)
        n199 = Or(x=w481, y=w480) -> (x .or. y?=w479:bool)
        n200 = Select(t=w469, s=w479, f=w471) -> (s? t:f=w478:string)
      }
      event "+": Mouse Down {
        w510 = "+"
        # "當前面已有運算子時\n不重複輸入+號"
        # "有錯誤訊息時不能輸入"
        n201 = event-data() -> ()  [unwired: 1 in, 8 out]
        n202 = Not Equal To 0?(x=w517) -> (x != 0?=w516:bool)
        n203 = Match Pattern(string=w506, regular expression="=") -> (before substring=w504:string)  [unwired: 1 in, 3 out]
        n204 = Equal?(x=w512, y=5) -> (x = y?=w511:bool)
        n205 = Concatenate Strings(w504, w510) -> (w509:string)
        n206 = Concatenate Strings(w506, w510) -> (w515:string)
        n207 = Select(t=w506, s=w516, f=w515) -> (s? t:f=w508:string)
        n208 = Select(t=w509, s=w511, f=w508) -> (s? t:f=w507:string)
        n209 = String Subset(string=w506, offset (0)=0, length (rest)=2) -> (substring=w522:string)
        n210 = Equal?(x="無", y=w522) -> (x = y?=w521:bool)
        n211 = Equal?(x=w522, y="輸") -> (x = y?=w520:bool)
        n212 = Or(x=w521, y=w520) -> (x .or. y?=w519:bool)
        n213 = Select(t=w506, s=w519, f=w507) -> (s? t:f=w518:string)
      }
      event "-": Mouse Down {
        w543 = "-"
        # "當前面已有運算子時\n不重複輸入-號"
        # "有錯誤訊息時不能輸入"
        n214 = event-data() -> ()  [unwired: 1 in, 8 out]
        n215 = Not Equal To 0?(x=w550) -> (x != 0?=w549:bool)
        n216 = Match Pattern(string=w539, regular expression="=") -> (before substring=w537:string)  [unwired: 1 in, 3 out]
        n217 = Equal?(x=w545, y=5) -> (x = y?=w544:bool)
        n218 = Concatenate Strings(w537, w543) -> (w542:string)
        n219 = Concatenate Strings(w539, w543) -> (w548:string)
        n220 = Select(t=w539, s=w549, f=w548) -> (s? t:f=w541:string)
        n221 = Select(t=w542, s=w544, f=w541) -> (s? t:f=w540:string)
        n222 = String Subset(string=w539, offset (0)=0, length (rest)=2) -> (substring=w555:string)
        n223 = Equal?(x="無", y=w555) -> (x = y?=w554:bool)
        n224 = Equal?(x=w555, y="輸") -> (x = y?=w553:bool)
        n225 = Or(x=w554, y=w553) -> (x .or. y?=w552:bool)
        n226 = Select(t=w539, s=w552, f=w540) -> (s? t:f=w551:string)
      }
      event "*": Mouse Down {
        w576 = "*"
        # "當前面已有運算子時\n不重複輸入*號"
        # "有錯誤訊息時不能輸入"
        n227 = event-data() -> ()  [unwired: 1 in, 8 out]
        n228 = Not Equal To 0?(x=w583) -> (x != 0?=w582:bool)
        n229 = Match Pattern(string=w572, regular expression="=") -> (before substring=w570:string)  [unwired: 1 in, 3 out]
        n230 = Equal?(x=w578, y=5) -> (x = y?=w577:bool)
        n231 = Concatenate Strings(w570, w576) -> (w575:string)
        n232 = Concatenate Strings(w572, w576) -> (w581:string)
        n233 = Select(t=w572, s=w582, f=w581) -> (s? t:f=w574:string)
        n234 = Select(t=w575, s=w577, f=w574) -> (s? t:f=w573:string)
        n235 = String Subset(string=w572, offset (0)=0, length (rest)=2) -> (substring=w588:string)
        n236 = Equal?(x="無", y=w588) -> (x = y?=w587:bool)
        n237 = Equal?(x=w588, y="輸") -> (x = y?=w586:bool)
        n238 = Or(x=w587, y=w586) -> (x .or. y?=w585:bool)
        n239 = Select(t=w572, s=w585, f=w573) -> (s? t:f=w584:string)
      }
      event "/": Mouse Down {
        w609 = "/"
        # "當前面已有運算子時\n不重複輸入/號"
        # "有錯誤訊息時不能輸入"
        n240 = event-data() -> ()  [unwired: 1 in, 8 out]
        n241 = Not Equal To 0?(x=w616) -> (x != 0?=w615:bool)
        n242 = Match Pattern(string=w605, regular expression="=") -> (before substring=w603:string)  [unwired: 1 in, 3 out]
        n243 = Equal?(x=w611, y=5) -> (x = y?=w610:bool)
        n244 = Concatenate Strings(w603, w609) -> (w608:string)
        n245 = Concatenate Strings(w605, w609) -> (w614:string)
        n246 = Select(t=w605, s=w615, f=w614) -> (s? t:f=w607:string)
        n247 = Select(t=w608, s=w610, f=w607) -> (s? t:f=w606:string)
        n248 = String Subset(string=w605, offset (0)=0, length (rest)=2) -> (substring=w621:string)
        n249 = Equal?(x="無", y=w621) -> (x = y?=w620:bool)
        n250 = Equal?(x=w621, y="輸") -> (x = y?=w619:bool)
        n251 = Or(x=w620, y=w619) -> (x .or. y?=w618:bool)
        n252 = Select(t=w605, s=w618, f=w606) -> (s? t:f=w617:string)
      }
      event "1/x": Mouse Down {
        w643 = "1/"
        # "有錯誤訊息時不能輸入"
        n253 = event-data() -> ()  [unwired: 1 in, 8 out]
        n254 = Not Equal To 0?(x=w647) -> ()  [unwired: 1 out]
        n255 = Equal?(x=w644, y=5) -> (x = y?=w635:bool)
        n256 = Match Pattern(string=w640, regular expression="=") -> (before substring=w638:string)  [unwired: 1 in, 3 out]
        n257 = Concatenate Strings(w638, w643) -> (w642:string)
        n258 = Concatenate Strings(w640, w643) -> (w636:string)
        n259 = Select(t=w642, s=w635, f=w636) -> (s? t:f=w641:string)
        n260 = String Subset(string=w640, offset (0)=0, length (rest)=2) -> (substring=w652:string)
        n261 = Equal?(x="無", y=w652) -> (x = y?=w651:bool)
        n262 = Equal?(x=w652, y="輸") -> (x = y?=w650:bool)
        n263 = Or(x=w651, y=w650) -> (x .or. y?=w649:bool)
        n264 = Select(t=w640, s=w649, f=w641) -> (s? t:f=w648:string)
      }
      event "=": Mouse Down {
        w666 = FALSE
        # "當前面已有運算子時\n不重複輸=/號"
        # "有錯誤訊息時不能輸入"
        n265 = event-data() -> ()  [unwired: 1 in, 8 out]
        n266 = Not Equal To 0?(x=w673) -> (x != 0?=w672:bool)
        n267 = Concatenate Strings(w669, "=") -> (w671:string)
        n268 = call <vilib>:"Eval Formula String.vi"("formula"=w669) -> ("y value"=w667:dbl)  [unwired: 1 in, 1 out]
        n269 = Select(t=w669, s=w672, f=w671) -> (s? t:f=w670:string)
        n270 = String Subset(string=w669, offset (0)=0, length (rest)=2) -> (substring=w679:string)
        n271 = Equal?(x="無", y=w679) -> (x = y?=w678:bool)
        n272 = Equal?(x=w679, y="輸") -> (x = y?=w677:bool)
        n273 = Or(x=w678, y=w677) -> (x .or. y?=w676:bool)
        n274 = Select(t=w669, s=w676, f=w670) -> (s? t:f=w675:string)
      }
      event "Save 1": Mouse Down {
        n275 = event-data() -> ()  [unwired: 1 in, 8 out]
        "Save1" <- w691
      }
      event "Save 2": Mouse Down {
        n276 = event-data() -> ()  [unwired: 1 in, 8 out]
        "Save 2" <- w703
      }
      event "+/-": Mouse Down {
        # "當顯示屏只有0一個數字時\n鎖定輸入負數符號的功能"
        # "有錯誤訊息時不能輸入"
        # "當顯示屏只有一個數字且為0時\n不輸入負數符號"
        n277 = event-data() -> ()  [unwired: 1 in, 8 out]
        n278 = String Length(string=w724) -> (length=w751:i32)
        n279 = Equal?(x=w751, y=1) -> (x = y?=w749:bool)
        n280 = Equal?(x=w724, y="0") -> (x = y?=w748:bool)
        n281 = And(x=w749, y=w748) -> (x .and. y?=w728:bool)
        n282 = Number To Decimal String(number=w719) -> (decimal integer string=w718:string)  [unwired: 1 in]
        n283 = Concatenate Strings(w724, "(-") -> (w737:string)
        n284 = Equal?(x=w721, y=5) -> (x = y?=w720:bool)
        n285 = Concatenate Strings("(-", w718) -> (w717:string)
        n286 = Not(x=w736) -> (.not. x?=w738:bool)
        n287 = Select(t=w724, s=w736, f=w737) -> (s? t:f=w727:string)
        n288 = Select(t=w736, s=w728, f=w738) -> (s? t:f=w735:bool)
        n289 = Not Equal To 0?(x=w734) -> (x != 0?=w733:bool)
        n290 = Select(t=w724, s=w728, f=w727) -> (s? t:f=w716:string)
        n291 = Select(t=FALSE, s=w733, f=w735) -> (s? t:f=w732:bool)
        n292 = Select(t=w717, s=w720, f=w716) -> (s? t:f=w715:string)
        n293 = String Subset(string=w724, offset (0)=0, length (rest)=2) -> (substring=w743:string)
        n294 = Equal?(x="無", y=w743) -> (x = y?=w742:bool)
        n295 = Equal?(x=w743, y="輸") -> (x = y?=w741:bool)
        n296 = Or(x=w742, y=w741) -> (x .or. y?=w731:bool)
        n297 = Select(t=w724, s=w731, f=w715) -> (s? t:f=w740:string)
        n298 = Select(t=FALSE, s=w731, f=w732) -> (s? t:f=w729:bool)
      }
      event "Backspace": Mouse Down {
        w775 = FALSE
        w780 = "0"
        # "有錯誤訊息時不能清除"
        # "每次消除1個最後輸入的字元\n當只剩最後一個字元或有負數剩兩個字元時\n將顯示屏清除為0"
        n299 = event-data() -> ()  [unwired: 1 in, 8 out]
        n300 = String Length(string=w765) -> (length=w794:i32)
        n301 = String Length(string=w765) -> (length=w781:i32)
        n302 = Equal?(x=w794, y=2) -> (x = y?=w782:bool)
        n303 = Equal?(x=w781, y=1) -> (x = y?=w778:bool)
        n304 = Decrement(x=w781) -> (x-1=w767:i32)
        n305 = And(x=w774, y=w782) -> (x .and. y?=w777:bool)
        n306 = String Subset(string=w765, offset (0)=0, length (rest)=w767) -> (substring=w764:string)
        n307 = Or(x=w778, y=w777) -> (x .or. y?=w776:bool)
        n308 = Select(t=w780, s=w778, f=w764) -> (s? t:f=w784:string)
        n309 = Select(t=w780, s=w777, f=w784) -> (s? t:f=w763:string)
        n310 = String Subset(string=w765, offset (0)=0, length (rest)=2) -> (substring=w788:string)
        n311 = Equal?(x="無", y=w788) -> (x = y?=w787:bool)
        n312 = Equal?(x=w788, y="輸") -> (x = y?=w786:bool)
        n313 = Or(x=w787, y=w786) -> (x .or. y?=w771:bool)
        n314 = Select(t=w765, s=w771, f=w763) -> (s? t:f=w785:string)
        n315 = Select(t=w775, s=w776, f=w774) -> (s? t:f=w773:bool)
        n316 = Select(t=w775, s=w776, f=w770) -> (s? t:f=w772:bool)
        n317 = Select(t=w770, s=w771, f=w772) -> (s? t:f=w769:bool)
        n318 = Select(t=w774, s=w771, f=w773) -> (s? t:f=w768:bool)
      }
      event ".": Mouse Down {
        # "當已有小數點時\n不能再輸入小數點\n否則插入字串後面"
        # "當前面為運算子時\n小數點已0.方式顯示"
        # "有錯誤訊息時不能輸入"
        n319 = event-data() -> ()  [unwired: 1 in, 8 out]
        n320 = Not Equal To 0?(x=w819) -> (x != 0?=w811:bool)
        n321 = Concatenate Strings(w802, ".") -> (w808:string)
        n322 = Select(t=w802, s=w810, f=w808) -> (s? t:f=w807:string)
        n323 = Equal?(x=w815, y=5) -> (x = y?=w813:bool)
        n324 = Match Pattern(string=w802, regular expression="=") -> (before substring=w801:string)  [unwired: 1 in, 3 out]
        n325 = Concatenate Strings(w802, "0.") -> (w817:string)
        n326 = Select(t=w817, s=w811, f=w807) -> (s? t:f=w806:string)
        n327 = String Subset(string=w802, offset (0)=0, length (rest)=2) -> (substring=w827:string)
        n328 = Concatenate Strings(w801, ".") -> (w805:string)
        n329 = Equal?(x="無", y=w827) -> (x = y?=w826:bool)
        n330 = Equal?(x=w827, y="輸") -> (x = y?=w825:bool)
        n331 = Select(t=w805, s=w813, f=w806) -> (s? t:f=w812:string)
        n332 = Or(x=w826, y=w825) -> (x .or. y?=w821:bool)
        n333 = Select(t=w802, s=w821, f=w812) -> (s? t:f=w824:string)
        n334 = Select(t=FALSE, s=w821, f=TRUE) -> (s? t:f=w820:bool)
      }
      event "CE": Mouse Down {
        w840 = 0
        w848 = FALSE
        # "清除顯示屏為0"
        n335 = event-data() -> ()  [unwired: 1 in, 8 out]
      }
      event "C": Mouse Down {
        w857 = 0.0
        w862 = 0
        w865 = FALSE
        # "使用者按確認後執行清除\n按否則保持原樣"
        # "清除計算數值記憶"
        # "清除計算功能記憶狀態"
        # "取消小數點和正負號記憶"
        # "清除顯示屏為0"
        n336 = event-data() -> ()  [unwired: 1 in, 8 out]
        n337 = call "Display Message to User"() -> ("Yes"=w851:bool)  [unwired: 10 in, 1 out]
        n338 = Select(t=w862, s=w851, f=w860) -> (s? t:f=w858:i32)
        n339 = Select(t=w865, s=w851, f=w867) -> (s? t:f=w866:bool)
        n340 = Select(t=w865, s=w851, f=w864) -> (s? t:f=w863:bool)
        n341 = Select(t=w857, s=w851, f=w856) -> (s? t:f=w854:dbl)
        n342 = Select(t=w857, s=w851, f=w855) -> (s? t:f=w850:dbl)
        n343 = Select(t=0, s=w851, f=w853) -> (s? t:f=w852:i32)
        n344 = Select(t="0", s=w851, f=w869) -> (s? t:f=w868:string)
        n345 = Select(t=w862, s=w851, f=w861) -> (s? t:f=w859:i32)
      }
      event "SQRT": Mouse Down {
        w885 = 0
        # "當按過=號後馬上按sqrt\n則不作用"
        # "如果只有0一個數字則替換0"
        # "有錯誤訊息不能輸入"
        # "當要開根號的數字為負數時\n跳出錯誤訊息"
        n346 = event-data() -> ()  [unwired: 1 in, 8 out]
        n347 = String Length(string=w881) -> (length=w892:i32)
        n348 = Equal?(x=w892, y=1) -> (x = y?=w889:bool)
        n349 = Equal?(x=w881, y="0") -> (x = y?=w888:bool)
        n350 = Match Pattern(string=w881, regular expression="=") -> (before substring=w875:string)  [unwired: 1 in, 3 out]
        n351 = And(x=w889, y=w888) -> (x .and. y?=w886:bool)
        n352 = Concatenate Strings(w881, "sqrt(") -> (w887:string)
        n353 = Equal?(x=w883, y=5) -> (x = y?=w882:bool)
        n354 = Select(t="sqrt(", s=w886, f=w887) -> (s? t:f=w879:string)
        n355 = Select(t=w875, s=w882, f=w879) -> (s? t:f=w878:string)
        n356 = String Subset(string=w881, offset (0)=0, length (rest)=2) -> (substring=w904:string)
        n357 = Equal?(x="無", y=w904) -> (x = y?=w901:bool)
        n358 = Equal?(x=w904, y="輸") -> (x = y?=w900:bool)
        n359 = Or(x=w901, y=w900) -> (x .or. y?=w897:bool)
        n360 = Select(t="輸入的函數不正確", s=w895, f=w878) -> (s? t:f=w898:string)
        n361 = Select(t=w881, s=w897, f=w898) -> (s? t:f=w893:string)
      }
      event "stop": Mouse Down {
        n362 = event-data() -> ()  [unwired: 1 in, 8 out]
        n363 = Not(x="stop") -> (.not. x?=w913:bool)
      }
    }
    n364 = Subtract(x=w19, y=w20) -> (x-y=w17:u32)
    n365 = Divide(x=w17, y=1000) -> (x/y=w13:dbl)
    n366 = Number To Decimal String(number=w13) -> (decimal integer string=w14:string)  [unwired: 1 in]
    n367 = Concatenate Strings(w14, " s") -> (→"運行時間":string)
    n368 = Wait (ms)(milliseconds to wait=200) -> ()  [unwired: 1 out]
    "Display" <- w24
    "Answer" <- w11
  }
